vi "Byte Buffer.Mapping.Create (Block Reference).vi"(8 "error in (no error)":errorcluster, 9 "data type":T3, 10 "buffer offset":i32, 11 "Block Data Ref":T1 {"Data Reference" format="%.0x"}) -> (0 "error out":errorcluster, 2 "new buffer offset":i32, 3 "mapping":T4)   [LabVIEW 2016, in "VeriStand Data.lvlib" / "Byte Buffer.lvclass"]
uses:
  Byte Buffer.lvclass
  Byte Buffer.Mapping.ctl
  Typedefs/Typedefs.Data Types.ctl
  <vilib>/NI Veristand/Custom Device API/Block Data Reference.ctl
  <vilib>/NI Veristand/Custom Device API/Data Reference.ctl
  Data Channels/Channels.Inline.Data Reference to Pointer.vi
  Utilities/Utilities.Sizeof.Scalar.vi
  Data Channels/Channels.Inline.Reference Error Handler.vi
  <vilib>/NI Veristand/Custom Device API/Global Data Refs.vi
  VeriStand Data.lvlib
  <vilib>/NI Veristand/Custom Device API/Custom Device API.lvlib
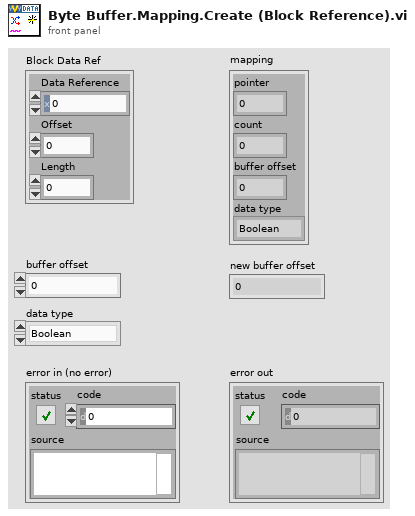
[diagram p1: front panel]
types:
  T1 = typedef "Custom Device API.lvlib/Block Data Reference.ctl" = cluster{"Data Reference":T2, "Offset":u64, "Length":u64}
  T2 = typedef "Custom Device API.lvlib/Data Reference.ctl" = i32
  T3 = typedef "VeriStand Data.lvlib/Typedefs.Data Types.ctl" = enum16{"Boolean", "Single", "Double", "I8", "I16", "I32", "I64", "U8", "U16", "U32", "U64"}
  T4 = typedef "VeriStand Data.lvlib/Byte Buffer.lvclass/Byte Buffer.Mapping.ctl" = cluster{"pointer":u64, "count":i32, "buffer offset":i32, "data type":T3}
  T5 = typedef "VeriStand Data.lvlib/Typedefs.Block Descriptor.Channel Block.ctl" = cluster{"block descriptor":T6, "offset":u64}
  T6 = typedef "VeriStand Data.lvlib/Typedefs.Block Descriptor.ctl" = cluster{"pointer":u64, "size":u64}
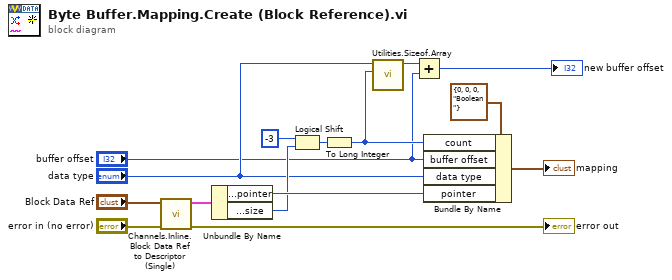
[diagram p0: block diagram]
diagram:
  n1 = call "Channels.Inline.Block Data Ref to Descriptor (Single).vi"("error in (no error)"="error in (no error)", "Block Data Ref"="Block Data Ref") -> ("error out"=→"error out":errorcluster, "Channel Block Descriptor"=w10:T5)  [unwired: 8 in]
  n2 = Unbundle By Name(w10) -> ("block descriptor.pointer"=w9:u64, "block descriptor.size"=w7:u64)
  n3 = Logical Shift(y=i16 -3, x=w7) -> (x << y=w8:u64)
  n4 = To Long Integer(number=w8) -> (32bit integer=w2:i32)
  n5 = call "Utilities.Sizeof.Array.vi"("count"=w2, "data type"="data type") -> ("size"=w5:u64)  [unwired: 9 in]
  n6 = Add(x=w5, y="buffer offset") -> (x+y=→"new buffer offset":u64)
  n7 = Bundle By Name(cluster=T4 {"pointer"=0, "count"=0, "buffer offset"=0, "data type"=enum."Boolean"} ("mapping"), "count"=w2, "buffer offset"="buffer offset", "data type"="data type", "pointer"=w9) -> (→"mapping":T4)
